vi "test14.1-MappingRelationshipByExternalRegistration_State.vi"() -> ()   [LabVIEW 2017, in "testcase-CSMBroadcast.lvclass"]
uses:
  testcase-CSMBroadcast.lvclass
  src/user.lib/_NEVSTOP/Communicable State Machine(CSM)/AdvanceAPI/CSM - Revert Arguments-Safe String.vi
  src/user.lib/_NEVSTOP/Communicable State Machine(CSM)/AdvanceAPI/CSM - Make String Arguments Safe.vi
  src/user.lib/_NEVSTOP/Communicable State Machine(CSM)/AdvanceAPI/CSM - Break Down Multiple States String.vi
  src/user.lib/_NEVSTOP/Communicable State Machine(CSM)/AdvanceAPI/CSM - Compact Multiple States.vi
  src/user.lib/_NEVSTOP/Communicable State Machine(CSM)/AdvanceAPI/CSM - Keywords.vi
  src/user.lib/_NEVSTOP/Communicable State Machine(CSM)/_Polymophic/CSM - Replace Marks in Messages.vi
  src/user.lib/_NEVSTOP/Communicable State Machine(CSM)/_Shared/Trim Single-line Text.vi
  src/user.lib/_NEVSTOP/Communicable State Machine(CSM)/Communicable State Machine.lvlib
  <vilib>/addons/_JKI Toolkits/VI Tester/TestCase.llb/TestCase.lvclass
  C:/Program Files (x86)/National Instruments/LabVIEW 2017/vi.lib/addons/_JKI Toolkits/VI Tester/TestCase.llb/TestCase.lvclass
panel:
  out "State History":string
  out "Rules 3":T1(array[cluster])
  out "Status In Registry 3":string[](array[string])
  out "Rules 4":T1(array[cluster])
  out "Status In Registry 4":string[](array[string])
  out "Loop Count 2":i32
  out "Error Array 2":errorcluster[](array[cluster])
  out "TestCase out":refnum<class "testcase-CSMBroadcast.lvclass">
  in  "TestCase in":refnum<class "testcase-CSMBroadcast.lvclass">
  out "error out":errorcluster
  in  "error in (no error)":errorcluster
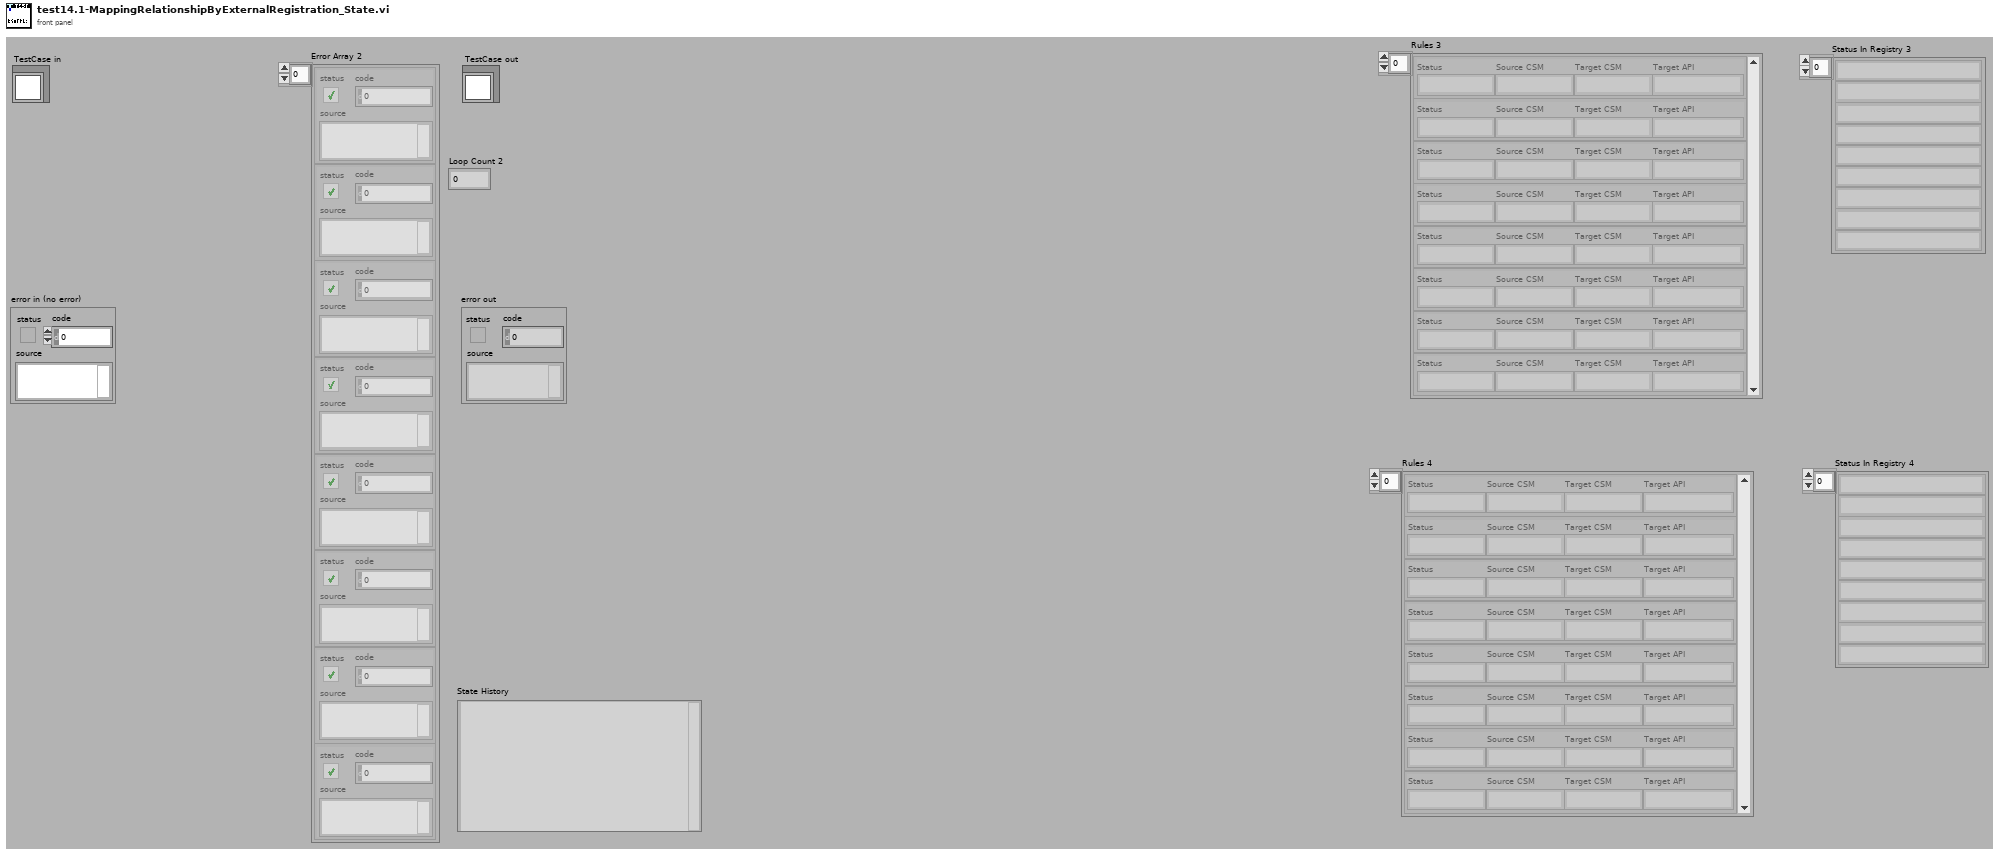
[diagram p1: front panel]
types:
  T1 = cluster{"Status":string, "Source CSM":string, "Target CSM":string, "Target API":string}[]
  T2 = enum32{"Invalid", "Standard", "Closed", "Hidden", "Minimized", "Maximized"}
  T3 = enum32{"invalid app kind", "Development System", "Run Time System", "Student Edition", "Embedded LabVIEW", "Evaluation", "Custom"}
  T4 = typedef "Communicable State Machine.lvlib/_CSM_Response Source Message.ctl" = cluster{"‘State":string, "’Arguments":string, "’Error":errorcluster}
  T5 = cluster{"Current VI Reference":refnum<vi>, "Close Panel on Exit?":bool}
  T6 = cluster{"Core":cluster{"Current VI Reference":refnum<vi>, "Close Panel on Exit?":bool}, "Your Boolean data":bool, "Your string data":string}
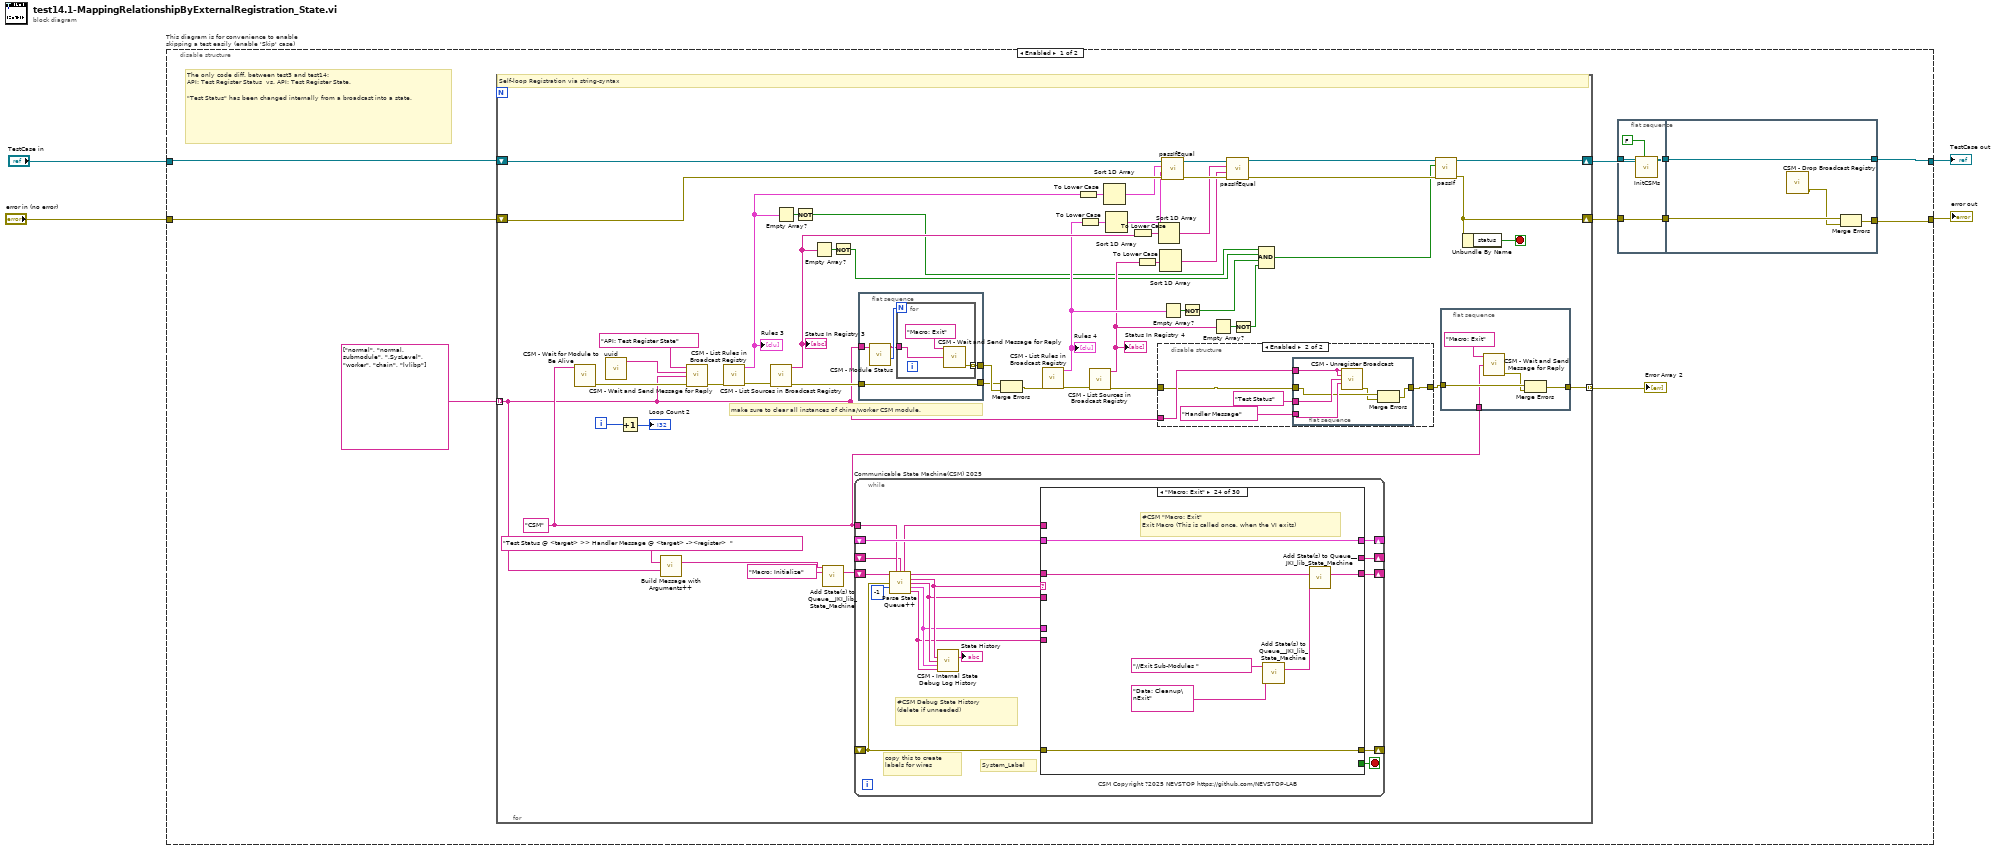
[diagram p0: block diagram]
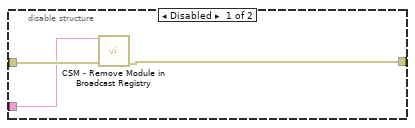
[diagram p2: hidden frame]
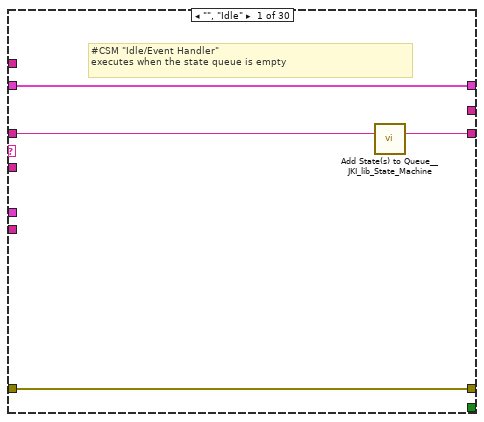
[diagram p3: hidden frame]
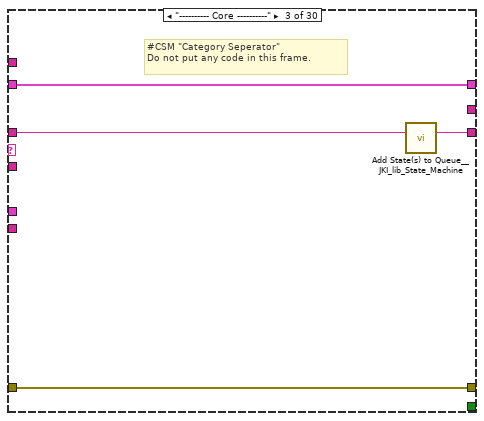
[diagram p5: hidden frame]
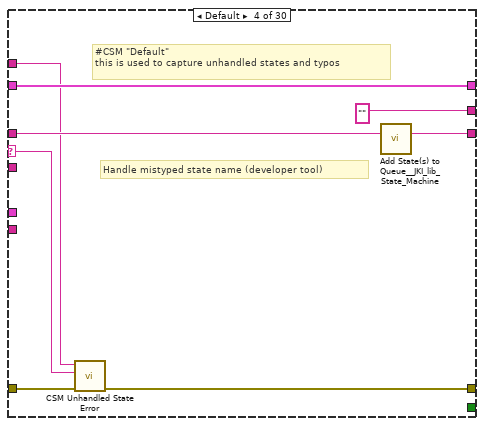
[diagram p6: hidden frame]
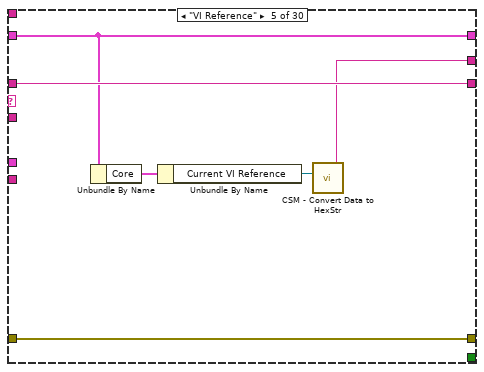
[diagram p7: hidden frame]
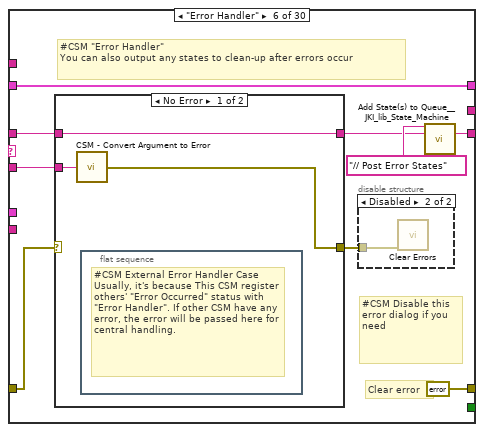
[diagram p8: hidden frame]
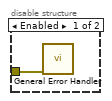
[diagram p9: hidden frame]
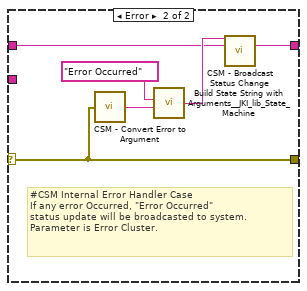
[diagram p10: hidden frame]
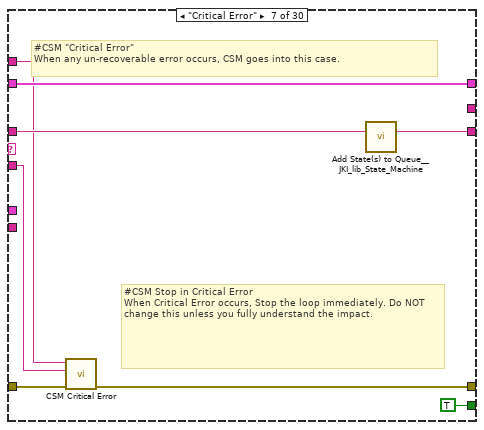
[diagram p11: hidden frame]
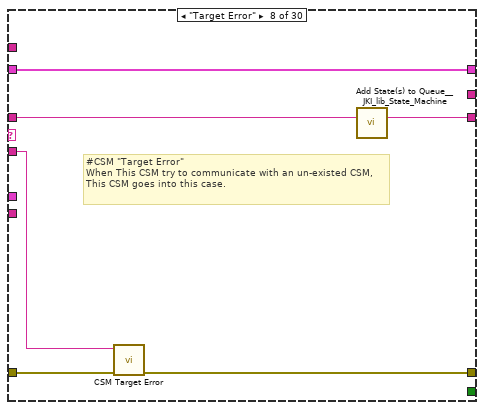
[diagram p12: hidden frame]
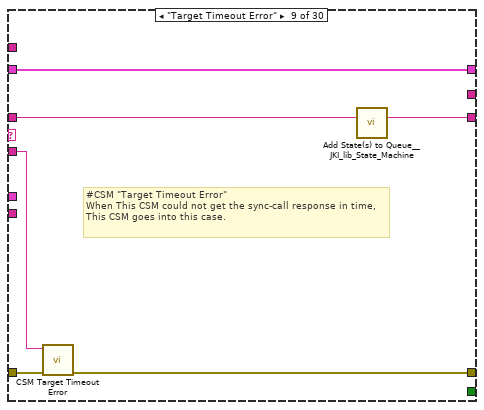
[diagram p13: hidden frame]
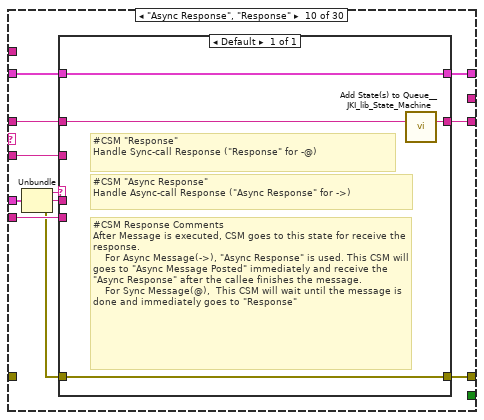
[diagram p14: hidden frame]
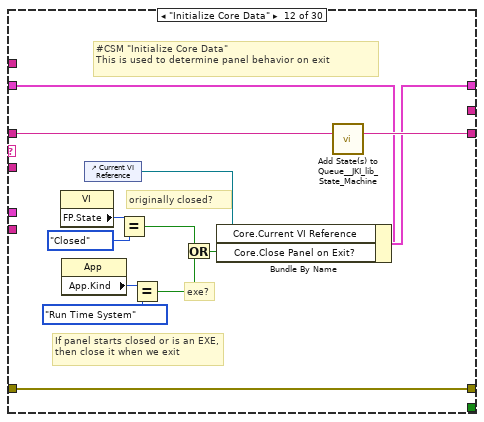
[diagram p16: hidden frame]
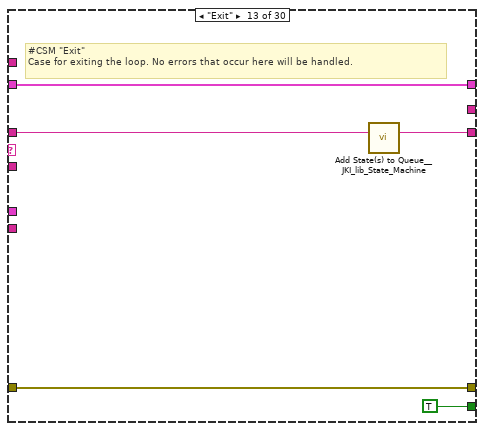
[diagram p17: hidden frame]
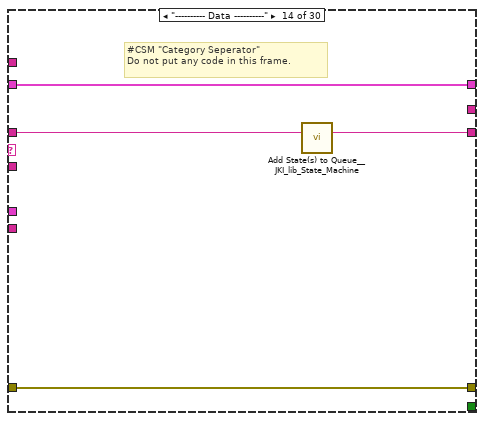
[diagram p18: hidden frame]
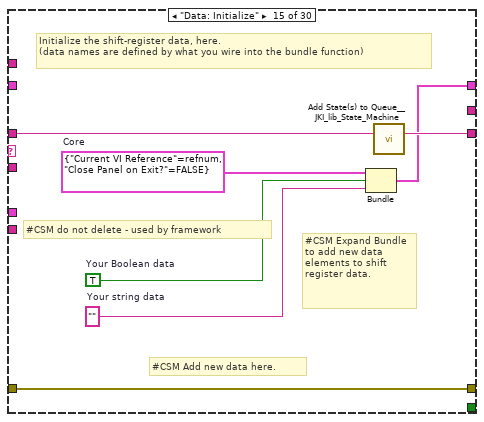
[diagram p19: hidden frame]
diagram:
  n1 = disable-structure "This diagram is for convenience to enable skipping a test easily (enable 'Skip' case)" shown="Enabled" {
    disable-tunnel: "TestCase in" -> [w6 w379]
    disable-tunnel: [w13 w377] -> w1
    disable-tunnel: [w7 w378] -> w3
    disable-tunnel: "error in (no error)" -> [w5 w376]
    frame Enabled {
      # "The only code diff. between test3 and test14:\nAPI: Test Register Status  vs. API: Test Register State.\n\n\"Test Status\" has been changed internally from a broadcast into a state."
      n2 = for {
        tunnel: string[] ["normal", "normal.submodule", ".SysLevel", "worker", "chain", "lvlibp"] -> [w23] mode=indexing
        shift-right: [w38] -> w14
        shift-left: w6 -> [w68]
        shift-right: [w36] -> w8
        shift-left: w5 -> [w67]
        tunnel: [w31] -> w12 mode=indexing
        i -> [w53]
        stop <- w66 stop-if-true
        w30 = "CSM" ("Name (\"\" to Use UUID)")
        # "make sure to clear all instances of china/worker CSM module."
        # "Self-loop Registration via string-syntax"
        n3 = call "CSM - Wait for Module to Be Alive.vi"("CSM Name"=w30) -> ("error out"=w29:errorcluster)  [unwired: 12 in, 2 out]
        n4 = call "uuid.vi"() -> ("UUID"=w72:string)  [unwired: 11 in]
        n5 = Increment(x=w53) -> (x+1=→"Loop Count 2":i32)
        n6 = call-poly "Build Message with Arguments++.vi"("States With Replace Token"="Test Status @ <target> >> Handler Message @ <target> -><register>  " ("State"), "<target>"=w23) -> ("States"=w26:string)  [unwired: 13 in]
        n7 = call "CSM - Wait and Send Message for Reply.vi"("State"="API: Test Register State", "Arguments (\"\")"=w72, "Target Module"=w23, "Error In (No Error)"=w29) -> ("error out"=w71:errorcluster)  [unwired: 9 in, 2 out]
        n8 = call "CSM - List Rules in Broadcast Registry.vi"("error in (no error)"=w71) -> ("error out"=w65:errorcluster, "Rule Entries"=w49:T1)  [unwired: 8 in, 1 out]
        "Rules 3" <- w49
        n9 = call "CSM - List Sources in Broadcast Registry.vi"("error in (no error)"=w65) -> ("error out"=w51:errorcluster, "Broadcast Names"=w46:string[])  [unwired: 9 in]
        "Status In Registry 3" <- w46
        n10 = Empty Array?(array=w49) -> (empty?=w48:bool)
        n11 = Not(x=w48) -> (.not. x?=w41:bool)
        n12 = Empty Array?(array=w46) -> (empty?=w47:bool)
        n13 = call <vilib>:"Add State(s) to Queue__JKI_lib_State_Machine.vi"("State(s) in Front (\"\")"=w26, "State(s) in (\"\")"="Macro: Initialize" ("Init State(\"Macro: Initialize\")")) -> ("States Out"=w27:string)  [unwired: 13 in]
        n14 = Not(x=w47) -> (.not. x?=w40:bool)
        n15 = while "Communicable State Machine(CSM) 2025" {
          shift-right: [w105] -> _
          shift-left: _ -> [w104]
          shift-right: [w108] -> _
          shift-left: _ -> [w103]
          shift-right: [w107] -> _
          shift-left: w27 -> [w109]
          tunnel: w30 -> [w101]
          shift-right: [w102] -> _
          shift-left: _ -> [w95]
          stop <- w106 stop-if-true
          # "#CSM Debug State History\n(delete if unneeded)"
          # "copy this to create labels for wires"
          # "System_Label"
          # "CSM Copyright ?2025 NEVSTOP https://github.com/NEVSTOP-LAB"
          n16 = call "Parse State Queue++.vi"("State Queue"=w109, "Name (\"\" to Use UUID)"=w101, "Response Arguments"=w95, "Previous Error"=w103, "Dequeue (1 ms)"=-1 ("Timeout")) -> ("Name Used"=w96:string, "Remaining States"=w110:string, "Current State"=w100:string, "Arguments"=w99:string, "Additional Information"=w98:T4, "Source CSM"=w97:string)  [unwired: 5 in]
          n17 = call "CSM - Internal State Debug Log History.vi"("State"=w100, "Arguments (\"\")"=w99, ">> Response Source Message >>"=w98, "Source (\"\")"=w97) -> ("Debug Log"=→"State History":string)  [unwired: 11 in]
          n18 = case shown="\"Macro: Exit\"" w100 {
            selector: w100 -> [_ _ _ w124 _ _ _ _ _ _ _ _ _ _ _ _ _ _ _ _ _ _ _ _ _ _ _ _ _ _]
            tunnel: w110 -> [w111 w116 w121 w128 w134 w140 w161 w167 w173 w181 w192 w206 w211 w215 w222 w224 w231 w235 w239 w245 w260 w329 w334 w341 w343 w347 w352 w359 w363 w367]
            tunnel: w99 -> [_ _ _ _ _ w139 w157 w166 w171 w180 _ _ _ _ _ _ _ _ _ w240 w254 _ _ _ _ _ w350 _ _ _]
            tunnel: w104 -> [w112 w115 w118 w126 w133 w143 w162 w168 w174 w183 w191 w199 w209 w212 _ w223 w226 w232 w237 w243 w256 w326 w331 w338 w342 w346 w351 w356 w360 w364]
            tunnel: [w113 w117 w119 w122 w135 errorcluster {"status"=FALSE, "code"=0, "source"=""} ("error out") w158 w164 w170 w186 w193 w203 w208 w213 w219 w225 w227 w233 w236 w241 w257 w327 w332 w339 w344 w348 w353 w357 w361 w365] -> w108
            tunnel: w103 -> [w113 w117 w119 w129 w135 w141 w163 w165 w172 _ w193 w203 w208 w213 w219 w225 w228 w233 w236 w242 w258 w327 w332 w339 w344 w348 w353 w357 w361 w365]
            tunnel: [w114 w116 w120 w127 w134 w136 w160 w169 w175 w182 w192 w205 w210 w214 w221 w224 w230 w234 w238 w244 w259 w328 w333 w340 w343 w347 w352 w358 w362 w366] -> w107
            tunnel: [_ _ _ _ _ _ TRUE _ _ _ _ _ TRUE _ _ _ _ _ _ _ _ _ _ _ _ _ _ _ _ _] -> w106
            tunnel: [w112 w115 w118 w126 w133 w143 w162 w168 w174 w184 w191 w204 w209 w212 w220 w223 w226 w232 w237 w243 w256 w326 w331 w338 w342 w346 w351 w356 w360 w364] -> w105
            tunnel: w97 -> [_ _ _ _ _ _ _ _ _ w178 _ _ _ _ _ _ _ _ _ _ _ _ _ _ _ _ _ _ _ _]
            tunnel: w98 -> [_ _ _ _ _ _ _ _ _ w185 _ _ _ _ _ _ _ _ _ _ _ _ _ _ _ _ _ _ _ _]
            tunnel: [_ _ _ "" w130 _ _ _ _ _ _ _ _ _ _ _ _ _ _ _ _ _ _ _ _ "API1 Response" w349 _ _ _] -> w102
            tunnel: w96 -> [_ _ _ w123 _ _ w156 _ _ _ _ _ _ _ _ _ _ _ _ _ _ _ _ _ _ _ _ _ _ _]
            frame "", "Idle" {
              # "#CSM \"Idle/Event Handler\"\nexecutes when the state queue is empty"
              n19 = call <vilib>:"Add State(s) to Queue__JKI_lib_State_Machine.vi"("State(s) in (\"\")"=w111) -> ("States Out"=w114:string)  [unwired: 14 in]
            }
            frame "CSM Documentation" {
              # "#CSM README FIRST\n\nCommunicable State Machine(CSM) is a LabVIEW application framework that builds upon JKI State Machine(JKISM). It follows the pattern of JKISM and extends the keywords to describe message communication between modules, including concepts such as Sync-Message, Async-Message, Subscription/Unsubscription of status - essential elements for creating reusable code modules. For more information, please visit the CSM wiki: https://nevstop-lab.github.io/CSM-Wiki/\n\nFor instructions on JKI State Machine, visit: http://jki.net/state-machine/\nFor information about CSM, visit: https://github.com/NEVSTOP-LAB"
              # "#CSM \"Documentation\"\nCase for holding CSM Documenation"
            }
            frame "---------- Core ----------" {
              # "#CSM \"Category Seperator\"\nDo not put any code in this frame."
              n20 = call <vilib>:"Add State(s) to Queue__JKI_lib_State_Machine.vi"("State(s) in (\"\")"=w121) -> ("States Out"=w120:string)  [unwired: 14 in]
            }
            frame Default {
              # "#CSM \"Default\"\nthis is used to capture unhandled states and typos"
              # "Handle mistyped state name (developer tool)"
              n21 = call "CSM Unhandled State Error.vi"("error in (no error)"=w129, "Undefined State"=w124, "CSM Name"=w123) -> ("error out"=w122:errorcluster)  [unwired: 8 in]
              n22 = call <vilib>:"Add State(s) to Queue__JKI_lib_State_Machine.vi"("State(s) in (\"\")"=w128) -> ("States Out"=w127:string)  [unwired: 14 in]
            }
            frame "VI Reference" {
              n23 = Unbundle By Name(w133) -> ("Core"=w132:T5)
              n24 = Unbundle By Name(w132) -> ("Current VI Reference"=w131:refnum<vi>)
              n25 = call "CSM - Convert Data to HexStr.vi"("Variant"=w131) -> ("HEX String (0-9,A-F)"=w130:string)  [unwired: 8 in]
            }
            frame "Error Handler" {
              # "#CSM Disable this error dialog if you need"
              # "#CSM \"Error Handler\"\nYou can also output any states to clean-up after errors occur"
              # "Clear error"
              n26 = case shown="No Error" w141 {
                selector: w141 -> [_ w150]
                tunnel: [w149 w152] -> w137
                tunnel: w140 -> [w149 w151]
                tunnel: w139 -> [w148 _]
                tunnel: [w147 w150] -> w142
                frame No Error {
                  n27 = call "CSM - Convert Argument to Error.vi"("Argument"=w148) -> ("Error"=w147:errorcluster)  [unwired: 4 in]
                  n28 = flat-sequence {
                    frame #0 {
                      # "#CSM External Error Handler Case\nUsually, it's because This CSM register others' \"Error Occurred\" status with \"Error Handler\". If other CSM have any error, the error will be passed here for central handling."
                    }
                  }
                }
                frame Error {
                  # "#CSM Internal Error Handler Case \nIf any error Occurred, \"Error Occurred\" \nstatus update will be broadcasted to system.\nParameter is Error Cluster."
                  n29 = call "CSM - Convert Error to Argument.vi"("Error"=w150) -> ("Argument"=w154:string)  [unwired: 4 in]
                  n30 = call <vilib>:"Build State String with Arguments__JKI_lib_State_Machine.vi"("Arguments (\"\")"=w154, "State"="Error Occurred" ("Status with Arguments")) -> ("State with Arguments"=w153:string)  [unwired: 4 in]
                  n31 = call "CSM - Broadcast Status Change.vi"("Status With Arguments"=w153, "State Queue"=w151) -> ("Remaining States"=w152:string)  [unwired: 13 in]
                }
              }
              n32 = disable-structure shown="Disabled" {
                disable-tunnel: w142 -> [w145 w146]
                frame Enabled {
                  n33 = call <vilib>:"General Error Handler.vi"("error in (no error)"=w145) -> ()  [unwired: 10 in, 5 out]
                }
                frame Disabled {
                  n34 = call <vilib>:"Clear Errors.vi"("error in (no error)"=w146) -> ()  [unwired: 5 in, 2 out]
                }
              }
              n35 = call <vilib>:"Add State(s) to Queue__JKI_lib_State_Machine.vi"("State(s) in Front (\"\")"="// Post Error States", "State(s) in (\"\")"=w137) -> ("States Out"=w136:string)  [unwired: 13 in]
            }
            frame "Critical Error" {
              # "#CSM Stop in Critical Error\nWhen Critical Error occurs, Stop the loop immediately. Do NOT change this unless you fully understand the impact."
              # "#CSM \"Critical Error\"\nWhen any un-recoverable error occurs, CSM goes into this case."
              n36 = call "CSM Critical Error.vi"("error in (no error)"=w163, "Arugments (As Reason)"=w157, "CSM Name"=w156) -> ("error out"=w158:errorcluster)  [unwired: 8 in]
              n37 = call <vilib>:"Add State(s) to Queue__JKI_lib_State_Machine.vi"("State(s) in (\"\")"=w161) -> ("States Out"=w160:string)  [unwired: 14 in]
            }
            frame "Target Error" {
              # "#CSM \"Target Error\"\nWhen This CSM try to communicate with an un-existed CSM, This CSM goes into this case."
              n38 = call "CSM Target Error.vi"("error in (no error)"=w165, "Arguments (As CSM Name)"=w166) -> ("error out"=w164:errorcluster)  [unwired: 9 in]
              n39 = call <vilib>:"Add State(s) to Queue__JKI_lib_State_Machine.vi"("State(s) in (\"\")"=w167) -> ("States Out"=w169:string)  [unwired: 14 in]
            }
            frame "Target Timeout Error" {
              # "#CSM \"Target Timeout Error\"\nWhen This CSM could not get the sync-call response in time, This CSM goes into this case."
              n40 = call "CSM Target Timeout Error.vi"("error in (no error)"=w172, "Arguments (As CSM Name)"=w171) -> ("error out"=w170:errorcluster)  [unwired: 9 in]
              n41 = call <vilib>:"Add State(s) to Queue__JKI_lib_State_Machine.vi"("State(s) in (\"\")"=w173) -> ("States Out"=w175:string)  [unwired: 14 in]
            }
            frame "Async Response", "Response" {
              n42 = Unbundle(w185) -> ("‘State"=w179:string, "’Arguments"=w177:string, "’Error"=w176:errorcluster)
              n43 = case shown="Default" w179 {
                tunnel: [w190] -> w186
                tunnel: w176 -> [w190]
                tunnel: [w189] -> w184
                tunnel: w183 -> [w189]
                tunnel: [w187] -> w182
                tunnel: w181 -> [w188]
                tunnel: w180 -> [_]
                tunnel: w178 -> [_]
                tunnel: w177 -> [_]
                frame Default {
                  # "#CSM Response Comments\nAfter Message is executed, CSM goes to this state for receive the response.\n    For Async Message(->), \"Async Response\" is used. This CSM will goes to \"Async Message Posted\" immediately and receive the \"Async Response\" after the callee finishes the message.\n    For Sync Message(@),  This CSM will wait until the message is done and immediately goes to \"Response\""
                  # "#CSM \"Async Response\"\nHandle Async-call Response (\"Async Response\" for ->)"
                  # "#CSM \"Response\"\nHandle Sync-call Response (\"Response\" for -@)"
                  n44 = call <vilib>:"Add State(s) to Queue__JKI_lib_State_Machine.vi"("State(s) in (\"\")"=w188) -> ("States Out"=w187:string)  [unwired: 14 in]
                }
              }
            }
            frame "Async Message Posted" {
              # "#CSM \"Async Message Posted\"\nAfter Async Message is posted (-> or ->| ), CSM goes to this state for post-action.\nYou can use Argument - State to tell which Async Message is called."
            }
            frame "Initialize Core Data" {
              # "#CSM \"Initialize Core Data\"\nThis is used to determine panel behavior on exit"
              # "originally closed?"
              # "exe?"
              # "If panel starts closed or is an EXE, then close it when we exit"
              n45 = property class="VI"() -> ("FP.State"=w196:T2)  [unwired: 2 in, 2 out]
              n46 = property class="App"() -> ("App.Kind"=w202:T3)  [unwired: 2 in, 2 out]
              n47 = control-ref of="Current VI Reference"() -> (w197:refnum<vi>)
              n48 = Equal?(x=w196, y=T2."Closed" ("Front Panel Window:State")) -> (x = y?=w194:bool)
              n49 = Equal?(x=w202, y=T3."Run Time System" ("Application:Kind")) -> (x = y?=w200:bool)
              n50 = Or(x=w194, y=w200) -> (x .or. y?=w198:bool)
              n51 = Bundle By Name(cluster=w199, "Core.Current VI Reference"=w197, "Core.Close Panel on Exit?"=w198) -> (w204:T6)
              n52 = call <vilib>:"Add State(s) to Queue__JKI_lib_State_Machine.vi"("State(s) in (\"\")"=w206) -> ("States Out"=w205:string)  [unwired: 14 in]
            }
            frame "Exit" {
              # "#CSM \"Exit\"\nCase for exiting the loop. No errors that occur here will be handled."
              n53 = call <vilib>:"Add State(s) to Queue__JKI_lib_State_Machine.vi"("State(s) in (\"\")"=w211) -> ("States Out"=w210:string)  [unwired: 14 in]
            }
            frame "---------- Data ----------" {
              # "#CSM \"Category Seperator\"\nDo not put any code in this frame."
              n54 = call <vilib>:"Add State(s) to Queue__JKI_lib_State_Machine.vi"("State(s) in (\"\")"=w215) -> ("States Out"=w214:string)  [unwired: 14 in]
            }
            frame "Data: Initialize" {
              w216 = T5 {"Current VI Reference"=refnum, "Close Panel on Exit?"=FALSE}  # Core
              w218 = TRUE  # Your Boolean data
              w217 = ""  # Your string data
              # "#CSM do not delete - used by framework"
              # "#CSM Expand Bundle to add new data elements to shift register data."
              # "#CSM Add new data here."
              # "Initialize the shift-register data, here.\n(data names are defined by what you wire into the bundle function)"
              n55 = Bundle("Core"=w216, "Your Boolean data"=w218, "Your string data"=w217) -> (w220:T6)  [unwired: 1 in]
              n56 = call <vilib>:"Add State(s) to Queue__JKI_lib_State_Machine.vi"("State(s) in (\"\")"=w222) -> ("States Out"=w221:string)  [unwired: 14 in]
            }
            frame "Data: Update Indicators" {
            }
            frame "Data: Cleanup" {
              # "Cleanup any data and references, here.\n(this is called automatically, by the Macro: Exit)"
              n57 = Unbundle By Name(w226) -> ("Core.Current VI Reference"=w229:refnum<vi>)
              n58 = Close Reference(reference=w229, error in (no error)=w228) -> (error out=w227:errorcluster)
              n59 = call <vilib>:"Add State(s) to Queue__JKI_lib_State_Machine.vi"("State(s) in (\"\")"=w231) -> ("States Out"=w230:string)  [unwired: 14 in]
            }
            frame "---------- UI ----------" {
              # "#CSM \"Category Seperator\"\nDo not put any code in this frame."
              n60 = call <vilib>:"Add State(s) to Queue__JKI_lib_State_Machine.vi"("State(s) in (\"\")"=w235) -> ("States Out"=w234:string)  [unwired: 14 in]
            }
            frame "UI: Initialize" {
              # "#CSM \"UI: Initialize\"\nInitialize the User Interface, here.\n(this is called automatically, by the Macro: Init)"
              n61 = call <vilib>:"Add State(s) to Queue__JKI_lib_State_Machine.vi"("State(s) in (\"\")"=w239) -> ("States Out"=w238:string)  [unwired: 14 in]
            }
            frame "UI: Cursor Set" {
              # "#CSM \"UI: Cursor Set\"\nSet and Unset Cursor Busy.\n(Usage: \"UI: Cursor Set >> Busy|Idle\")"
              # "Argument"
              n62 = disable-structure shown="TARGET_TYPE!=Windows" {
                disable-tunnel: w242 -> [w248 w253]
                disable-tunnel: [w247 w253] -> w241
                disable-tunnel: w240 -> [w246 _]
                frame condition #0 (active) {
                  n63 = case shown="\"Idle\", Default" w246 {
                    tunnel: w248 -> [w250 w252]
                    tunnel: [w249 w251] -> w247
                    frame "Idle", Default {
                      n64 = call <vilib>:"Unset Busy.vi"("error in (no error)"=w250) -> ("error out"=w249:errorcluster)  [unwired: 10 in]
                    }
                    frame "Busy" {
                      n65 = call <vilib>:"Set Busy.vi"("error in (no error)"=w252) -> ("error out"=w251:errorcluster)  [unwired: 9 in, 1 out]
                    }
                  }
                }
                frame condition #1 {
                }
              }
              n66 = call <vilib>:"Add State(s) to Queue__JKI_lib_State_Machine.vi"("State(s) in (\"\")"=w245) -> ("States Out"=w244:string)  [unwired: 14 in]
            }
            frame "UI: Front Panel State" {
              # "#CSM \"UI: Front Panel State\"\nSet Front Panel Open or Closed\n(Usage: \"UI: Front Panel State >> Open|Close\")"
              # "Argument"
              n67 = Unbundle By Name(w256) -> ("Core.Current VI Reference"=w255:refnum<vi>)
              n68 = call <vilib>:"Add State(s) to Queue__JKI_lib_State_Machine.vi"("State(s) in (\"\")"=w260) -> ("States Out"=w259:string)  [unwired: 14 in]
              n69 = case shown="\"Close\", \"Closed\"" w254 {
                tunnel: w258 -> [w266 w281 w292 w305 w318]
                tunnel: [w268 w282 w294 w307 w320] -> w257
                tunnel: w255 -> [w267 w279 w293 w306 w319]
                frame "Open", "Standard", Default {
                  w261 = T2."Standard" ("State")
                  n70 = property class="VI"(reference=w267, error in=w266) -> (reference out=w264:refnum<vi>, error out=w265:errorcluster, "FP.State"=w263:T2)
                  n71 = Not Equal?(x=w263, y=w261) -> (x != y?=w262:bool)
                  n72 = case shown="True" w262 {
                    tunnel: [w272 w274] -> w268
                    tunnel: w265 -> [w271 w274]
                    tunnel: w264 -> [w270 _]
                    tunnel: w261 -> [w269 _]
                    frame True {
                      n73 = invoke class="VI" method="FP.Open"(reference=w270, error in=w271, "Activate"=TRUE, "State"=w269) -> (error out=w272:errorcluster)  [unwired: 1 in, 4 out]
                    }
                    frame False {
                    }
                  }
                }
                frame "Close", "Closed" {
                  n74 = property class="VI"(reference=w279, error in=w281) -> (reference out=w278:refnum<vi>, error out=w280:errorcluster, "FP.State"=w276:T2)
                  n75 = Not Equal?(x=w276, y=T2."Closed" ("Front Panel Window:State")) -> (x != y?=w275:bool)
                  n76 = case shown="False" w275 {
                    tunnel: [w283 w286] -> w282
                    tunnel: w280 -> [w283 w285]
                    tunnel: w278 -> [_ w284]
                    frame False {
                    }
                    frame True {
                      n77 = invoke class="VI" method="FP.Close"(reference=w284, error in=w285) -> (error out=w286:errorcluster)  [unwired: 1 in, 2 out]
                    }
                  }
                }
                frame "Hidden", "Hide" {
                  w287 = T2."Hidden" ("State")
                  n78 = property class="VI"(reference=w293, error in=w292) -> (reference out=w290:refnum<vi>, error out=w291:errorcluster, "FP.State"=w289:T2)
                  n79 = Not Equal?(x=w289, y=w287) -> (x != y?=w288:bool)
                  n80 = case shown="True" w288 {
                    tunnel: [w298 w299] -> w294
                    tunnel: w291 -> [w297 w299]
                    tunnel: w290 -> [w296 _]
                    tunnel: w287 -> [w295 _]
                    frame True {
                      n81 = invoke class="VI" method="FP.Open"(reference=w296, error in=w297, "State"=w295) -> (error out=w298:errorcluster)  [unwired: 2 in, 4 out]
                    }
                    frame False {
                    }
                  }
                }
                frame "Minimize", "Minimized" {
                  w300 = T2."Minimized" ("State")
                  n82 = property class="VI"(reference=w306, error in=w305) -> (reference out=w303:refnum<vi>, error out=w304:errorcluster, "FP.State"=w302:T2)
                  n83 = Not Equal?(x=w302, y=w300) -> (x != y?=w301:bool)
                  n84 = case shown="True" w301 {
                    tunnel: [w311 w312] -> w307
                    tunnel: w304 -> [w310 w312]
                    tunnel: w303 -> [w309 _]
                    tunnel: w300 -> [w308 _]
                    frame True {
                      n85 = invoke class="VI" method="FP.Open"(reference=w309, error in=w310, "State"=w308) -> (error out=w311:errorcluster)  [unwired: 2 in, 4 out]
                    }
                    frame False {
                    }
                  }
                }
                frame "Maximize", "Maximized" {
                  w313 = T2."Maximized" ("State")
                  n86 = property class="VI"(reference=w319, error in=w318) -> (reference out=w316:refnum<vi>, error out=w317:errorcluster, "FP.State"=w315:T2)
                  n87 = Not Equal?(x=w315, y=w313) -> (x != y?=w314:bool)
                  n88 = case shown="True" w314 {
                    tunnel: [w324 w325] -> w320
                    tunnel: w317 -> [w323 w325]
                    tunnel: w316 -> [w322 _]
                    tunnel: w313 -> [w321 _]
                    frame True {
                      n89 = invoke class="VI" method="FP.Open"(reference=w322, error in=w323, "State"=w321) -> (error out=w324:errorcluster)  [unwired: 2 in, 4 out]
                    }
                    frame False {
                    }
                  }
                }
              }
            }
            frame "---------- Macro ----------" {
              # "#CSM \"Category Seperator\"\nDo not put any code in this frame."
              n90 = call <vilib>:"Add State(s) to Queue__JKI_lib_State_Machine.vi"("State(s) in (\"\")"=w329) -> ("States Out"=w328:string)  [unwired: 14 in]
            }
            frame "Macro: Initialize" {
              # "#CSM \"Macro: Initialize\"\nInitialization Macro (This is called once, when the VI starts)"
              n91 = call <vilib>:"Add State(s) to Queue__JKI_lib_State_Machine.vi"("State(s) in Front (\"\")"="Data: Initialize\nInitialize Core Data\nData: Update Indicators", "State(s) in (\"\")"=w334) -> ("States Out"=w333:string)  [unwired: 13 in]
            }
            frame "Macro: Exit" {
              # "#CSM \"Macro: Exit\"\nExit Macro (This is called once, when the VI exits)"
              n92 = call <vilib>:"Add State(s) to Queue__JKI_lib_State_Machine.vi"("State(s) in Front (\"\")"="//Exit Sub-Modules ", "State(s) at Back (\"\")"="Data: Cleanup\nExit") -> ("States Out"=w336:string)  [unwired: 13 in]
              n93 = call <vilib>:"Add State(s) to Queue__JKI_lib_State_Machine.vi"("State(s) in Front (\"\")"=w336, "State(s) in (\"\")"=w341) -> ("States Out"=w340:string)  [unwired: 13 in]
            }
            frame "---------- API ----------" {
              # "#CSM \"Category Seperator\"\nDo not put any code in this frame."
            }
            frame "API: API1" {
              # "#CSM API Example\nCopy/Rename this case for your own API"
              # "#CSM Response\nConnect this to return the response of your API"
              # "#CSM >> Msg/Rep's CSM >>\nIf you need to tell who triggered this state , use this string. If it's this case itself, this string is \"\"."
              # "#CSM >> Arguments >>\nDeal with the parameter if any"
            }
            frame "API: API2" {
              # "#CSM API Example\nCopy/Rename this case for your own API"
              # "unpack Hex String  to Variant\nif complex parameter is needed."
              n94 = call "CSM - Convert HexStr to Data.vi"("HEX String"=w350) -> ()  [unwired: 7 in, 2 out]
              n95 = disable-structure shown="Disabled" {
                disable-tunnel: [w354 "API2 Response"] -> w349
                frame Disabled {
                  # "pack variant to hexstr \nif complex response is needed."
                  # "complex Response"
                  n96 = call "CSM - Convert Data to HexStr.vi"() -> ("HEX String (0-9,A-F)"=w354:string)  [unwired: 9 in]
                }
                frame Enabled {
                }
              }
            }
            frame "---------- Action ----------" {
              # "#CSM \"Category Seperator\"\nDo not put any code in this frame."
              n97 = call <vilib>:"Add State(s) to Queue__JKI_lib_State_Machine.vi"("State(s) in (\"\")"=w359) -> ("States Out"=w358:string)  [unwired: 14 in]
            }
            frame "Action: action1" {
              # "#CSM \"Internal State\"\nThis category is used for holding internal states"
              n98 = call <vilib>:"Add State(s) to Queue__JKI_lib_State_Machine.vi"("State(s) in (\"\")"=w363) -> ("States Out"=w362:string)  [unwired: 14 in]
            }
            frame "Action: action2" {
              # "#CSM \"Internal State\"\nThis category is used for holding internal states"
              n99 = call <vilib>:"Add State(s) to Queue__JKI_lib_State_Machine.vi"("State(s) in (\"\")"=w367) -> ("States Out"=w366:string)  [unwired: 14 in]
            }
          }
        }
        n100 = flat-sequence {
          tunnel: [w372] -> w70
          tunnel: w23 -> [w370]
          tunnel: [w369] -> w50
          tunnel: w51 -> [w369]
          frame #0 {
            n101 = call "CSM - Module Status.vi"("CSM Name"=w370) -> ("#Nodes"=w371:i32, "CSM Name (Dup)"=w368:string)  [unwired: 6 in, 3 out]
            n102 = for {
              N: w371 -> [_]
              tunnel: [w374] -> w372 mode=indexing
              tunnel: w368 -> [w373]
              n103 = call "CSM - Wait and Send Message for Reply.vi"("State"="Macro: Exit", "Target Module"=w373) -> ("error out"=w374:errorcluster)  [unwired: 11 in, 2 out]
            }
          }
        }
        n104 = Merge Errors(w50, w70) -> (w69:errorcluster)
        n105 = call "CSM - List Rules in Broadcast Registry.vi"("error in (no error)"=w69) -> ("error out"=w64:errorcluster, "Rule Entries"=w44:T1)  [unwired: 8 in, 1 out]
        "Rules 4" <- w44
        n106 = To Lower Case(string=w49) -> (all lower case string=w63:T1)
        n107 = To Lower Case(string=w44) -> (all lower case string=w62:T1)
        n108 = call "CSM - List Sources in Broadcast Registry.vi"("error in (no error)"=w64) -> ("error out"=w25:errorcluster, "Broadcast Names"=w42:string[])  [unwired: 9 in]
        "Status In Registry 4" <- w42
        n109 = Sort 1D Array(array=w63) -> (sorted array=w61:T1)
        n110 = Sort 1D Array(array=w62) -> (sorted array=w60:T1)
        n111 = To Lower Case(string=w46) -> (all lower case string=w57:string[])
        n112 = To Lower Case(string=w42) -> (all lower case string=w56:string[])
        n113 = disable-structure shown="Enabled" {
          disable-tunnel: w25 -> [w76 w80]
          disable-tunnel: w23 -> [w75 w81]
          disable-tunnel: [w74 w79] -> w24
          frame Disabled {
            n114 = call "CSM - Remove Module in Broadcast Registry.vi"("CSM Name"=w75, "Error In"=w76) -> ("error out"=w74:errorcluster)  [unwired: 12 in, 1 out]
          }
          frame Enabled {
            n115 = flat-sequence {
              tunnel: "Test Status" ("Status") -> [w87]
              tunnel: "Handler Message" ("Response Message (If \"\", Same as Source Message)") -> [w86]
              tunnel: w81 -> [w85]
              tunnel: w80 -> [w84]
              tunnel: [w82] -> w79
              frame #0 {
                n116 = call "CSM - Unregister Broadcast.vi"("CSM Name(Empty for Broadcast Event)"=w85, "Source CSM Name (* as Default)"=w85, "Trigger"=w87, "API (\"*\" as Default)"=w86) -> ("error out"=w83:errorcluster)  [unwired: 10 in, 1 out]
                n117 = Merge Errors(w84, w83) -> (w82:errorcluster)
              }
            }
          }
        }
        n118 = Sort 1D Array(array=w57) -> (sorted array=w55:string[])
        n119 = Sort 1D Array(array=w56) -> (sorted array=w54:string[])
        n120 = call-dynamic "passIfEqual.vi"("error in (no error)"=w67, "y"=w60, "x"=w61, "TestCase in"=w68) -> ("error out"=w58:errorcluster, "TestCase out"=w59:refnum<class "testcase-CSMBroadcast.lvclass">)  [unwired: 6 in]
        n121 = Empty Array?(array=w44) -> (empty?=w45:bool)
        n122 = Not(x=w45) -> (.not. x?=w34:bool)
        n123 = Empty Array?(array=w42) -> (empty?=w43:bool)
        n124 = call-dynamic "passIfEqual.vi"("error in (no error)"=w58, "y"=w54, "x"=w55, "TestCase in"=w59) -> ("error out"=w37:errorcluster, "TestCase out"=w39:refnum<class "testcase-CSMBroadcast.lvclass">)  [unwired: 6 in]
        n125 = Not(x=w43) -> (.not. x?=w33:bool)
        n126 = Compound Arithmetic op=AND(w41, w40, w34, w33) -> (w35:bool)
        n127 = call-dynamic "passIf.vi"("error in (no error)"=w37, "pass"=w35, "TestCase in"=w39) -> ("error out"=w36:errorcluster, "TestCase out"=w38:refnum<class "testcase-CSMBroadcast.lvclass">)  [unwired: 7 in]
        n128 = flat-sequence {
          tunnel: w24 -> [w91]
          tunnel: [w90] -> w31
          tunnel: w30 -> [w88]
          frame #0 {
            n129 = call "CSM - Wait and Send Message for Reply.vi"("State"="Macro: Exit", "Target Module"=w88) -> ("error out"=w89:errorcluster)  [unwired: 11 in, 2 out]
            n130 = Merge Errors(w91, w89) -> (w90:errorcluster)
          }
        }
        n131 = Unbundle By Name(w36) -> ("status"=w66:bool)
      }
      "Error Array 2" <- w12
      n132 = flat-sequence {
        tunnel: w14 -> [w18]
        tunnel: [w17] -> w10
        tunnel: [w16] -> w9
        tunnel: w8 -> [w16]
        tunnel: [w22] -> w13
        tunnel: w10 -> [w22]
        tunnel: w9 -> [w21]
        tunnel: [w20] -> w7
        frame #0 {
          n133 = call "InitCSMs.vi"("Enable building lvlibp?"=FALSE, "testcase-CSMStatus in"=w18) -> ("testcase-CSMStatus out"=w17:refnum<class "testcase-CSMBroadcast.lvclass">)  [unwired: 8 in, 1 out]
        }
        frame #1 {
          n134 = call "CSM - Drop Broadcast Registry.vi"() -> ("error out"=w19:errorcluster)  [unwired: 15 in]
          n135 = Merge Errors(w21, w19) -> (w20:errorcluster)
        }
      }
    }
    frame Disabled {
      # "skip test result while test is under development"
      n136 = call <vilib>:"skip.vi"("error in (no error)"=w376, "TestCase in"=w379) -> ("error out"=w378:errorcluster, "TestCase out"=w377:refnum<class "testcase-CSMBroadcast.lvclass">)  [unwired: 8 in]
    }
  }
  "error out" <- w3
  "TestCase out" <- w1
